vi "Drive Train Test.vi"(10 "Boolean":bool) -> ()   [LabVIEW 2018]
uses:
  SubSystems/Drive Train/Drive Train Global.vi
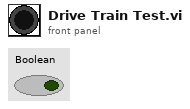
[diagram p1: front panel]
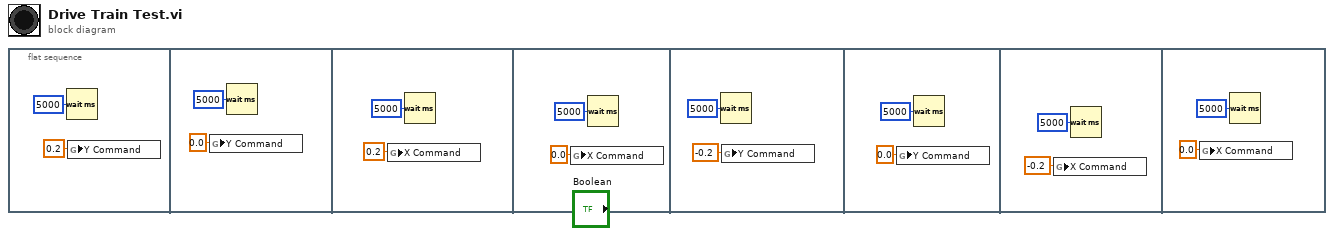
[diagram p0: block diagram]
diagram:
  n1 = flat-sequence {
    frame #0 {
      n2 = Wait (ms)(milliseconds to wait=u32 5000) -> ()  [unwired: 1 out]
      n3 = global write "Drive Train Global.vi" "Y Command"(0.2 ("Y Command")) -> ()
    }
    frame #1 {
      n4 = global write "Drive Train Global.vi" "Y Command"(0.0 ("Y Command")) -> ()
      n5 = Wait (ms)(milliseconds to wait=u32 5000) -> ()  [unwired: 1 out]
    }
    frame #2 {
      n6 = global write "Drive Train Global.vi" "X Command"(0.2 ("Y Command")) -> ()
      n7 = Wait (ms)(milliseconds to wait=u32 5000) -> ()  [unwired: 1 out]
    }
    frame #3 {
      n8 = global write "Drive Train Global.vi" "X Command"(0.0 ("Y Command")) -> ()
      n9 = Wait (ms)(milliseconds to wait=u32 5000) -> ()  [unwired: 1 out]
    }
    frame #4 {
      n10 = Wait (ms)(milliseconds to wait=u32 5000) -> ()  [unwired: 1 out]
      n11 = global write "Drive Train Global.vi" "Y Command"(-0.2 ("Y Command")) -> ()
    }
    frame #5 {
      n12 = global write "Drive Train Global.vi" "Y Command"(0.0 ("Y Command")) -> ()
      n13 = Wait (ms)(milliseconds to wait=u32 5000) -> ()  [unwired: 1 out]
    }
    frame #6 {
      n14 = global write "Drive Train Global.vi" "X Command"(-0.2 ("Y Command")) -> ()
      n15 = Wait (ms)(milliseconds to wait=u32 5000) -> ()  [unwired: 1 out]
    }
    frame #7 {
      n16 = global write "Drive Train Global.vi" "X Command"(0.0 ("Y Command")) -> ()
      n17 = Wait (ms)(milliseconds to wait=u32 5000) -> ()  [unwired: 1 out]
    }
  }
